vi "EOL Calculate Sunshade Data.vi"(8 "Truncation End":i32=15, 9 "Truncation Start":i32=15, 10 "Array Data":dbl[](array[numeric])) -> (0 "Current Out":dbl[](graph), 2 "Sunshade Data":dbl[](array[numeric]))   [LabVIEW 2018]
uses:
  <vilib>/Analysis/baseanly.llb/Mean (DBL).vi
  <vilib>/Analysis/NI_AALBase.lvlib
panel:
  out "Current Out 2":dbl[](graph)
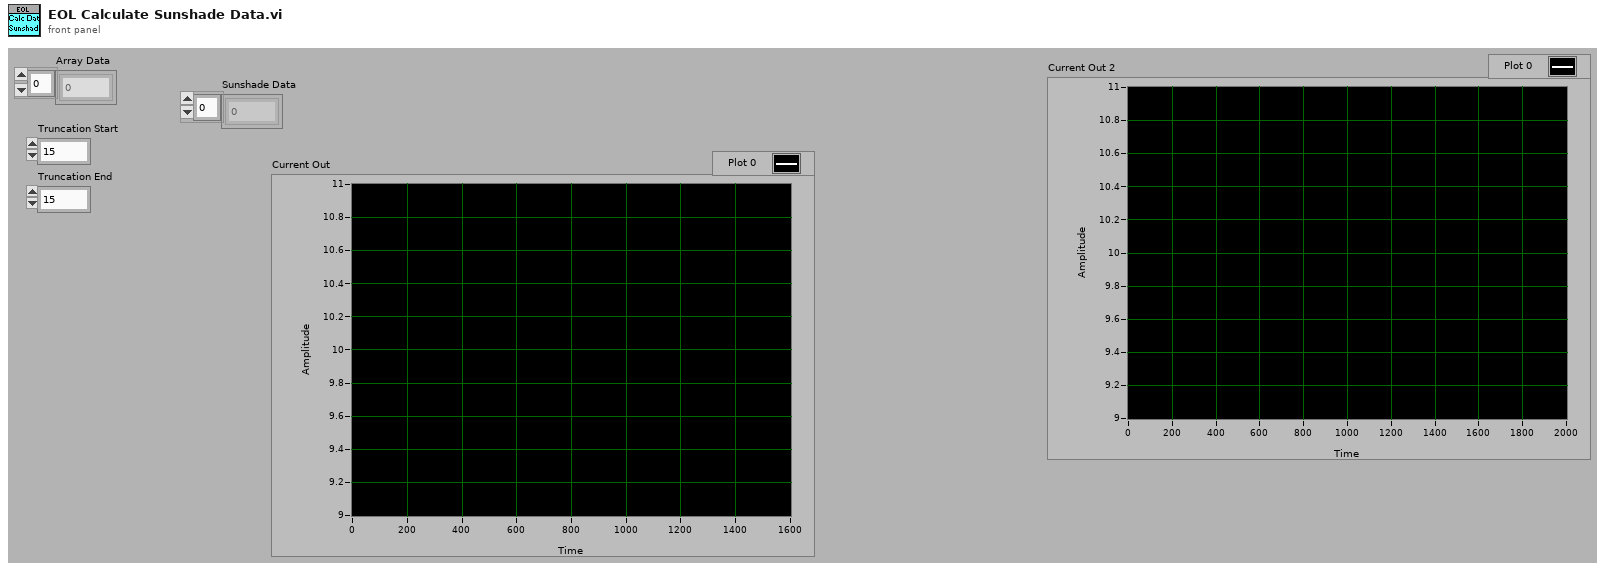
[diagram p1: front panel]
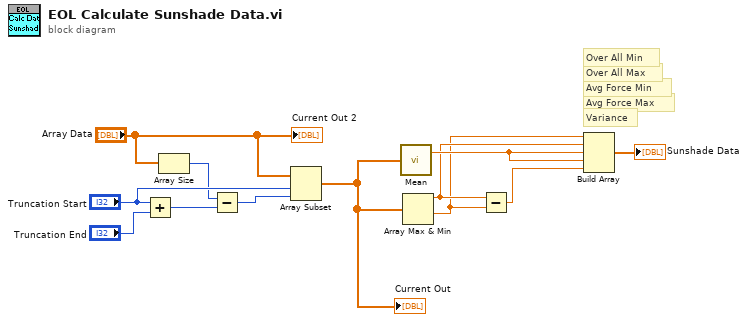
[diagram p0: block diagram]
diagram:
  # "Variance"
  # "Avg Force Max"
  # "Avg Force Min"
  # "Over All Max"
  # "Over All Min"
  n1 = Add(x="Truncation Start", y="Truncation End") -> (x+y=w9:i32)
  n2 = Array Size(array="Array Data") -> (size(s)=w10:i32)
  n3 = Subtract(x=w10, y=w9) -> (x-y=w8:i32)
  n4 = Array Subset(array="Array Data", index="Truncation Start", length=w8) -> (w2:dbl[])
  "Current Out" <- w2
  n5 = call-poly <vilib>:"Mean.vi"("X"=w2) -> ("mean"=w7:dbl)  [unwired: 1 out]
  n6 = Array Max & Min(array=w2) -> (max value=w5:dbl, min value=w4:dbl)  [unwired: 2 out]
  n7 = Subtract(x=w5, y=w4) -> (x-y=w6:dbl)
  n8 = Build Array(w4, w5, w7, w7, w6) -> (→"Sunshade Data":dbl[])
  "Current Out 2" <- "Array Data"
